vi "TelemetryServer_Disconnect.vi"(2 "Channel Name":string, 9 "error in (no error)":errorcluster caption="error out") -> (6 "error out":errorcluster)   [LabVIEW 2009]
uses:
  lib/lvrtc.dll
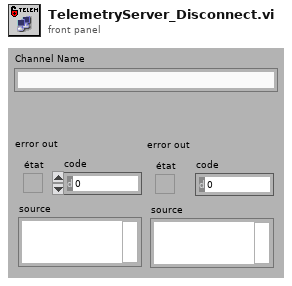
[diagram p1: front panel]
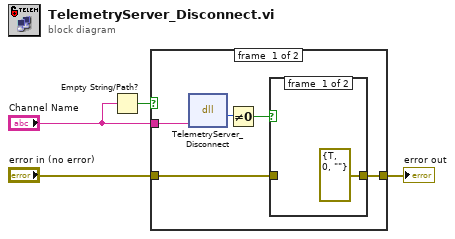
[diagram p0: block diagram]
diagram:
  n1 = Empty String/Path?(string/path="Channel Name") -> (empty?=w2:bool)
  n2 = case shown="False" w2 {
    tunnel: "Channel Name" -> [w9 _]
    tunnel: "error in (no error)" -> [w6 w12]
    tunnel: [w5 w12] -> w4
    frame #0 {
      n3 = dll-call lib="C:/Ohana/LV2009/OhanaOS-LV81/Instruments/RTC/Api/lib/lvrtc.dll" fn="TelemetryServer_Disconnect"("channelName"=w9) -> (w8:i32)  [unwired: 4 in, 2 out]
      n4 = Not Equal To 0?(x=w8) -> (x != 0?=w7:bool)
      n5 = case shown="True" w7 {
        tunnel: w6 -> [_ w11]
        tunnel: [errorcluster {"status"=TRUE, "code"=0, "source"=""} ("error in (no error)") w11] -> w5
        frame #0 {
        }
        frame #1 {
        }
      }
    }
    frame #1 {
    }
  }
  "error out" <- w4
